vi "Set Aout Cfactor.vi"(8 "error in (no error)":errorcluster, 9 "firmware revision":string(combo), 10 "aout cfactor":T2={"CFactorC (10.0)"=10.0, "CFactorL (100.0)"=100.0}, 11 "VISA resource name":refnum<visa-resource-name>) -> (0 "error out":errorcluster, 2 "bridge error":T1, 3 "VISA resource name out":refnum<visa-resource-name>)   [LabVIEW 2024, in "Andeen-Hagerling 2700A.lvlib"]
doc: "Sets the input to output voltage conversion factor for the\ncapacitance and loss voltage output channels in V/pF and\nV/jpF respectively. This VI gives a direct means of\ncontrolling the sensitivity of the voltage outputs to changes in\nthe DUT."
uses:
  Andeen-Hagerling 2700A.lvlib
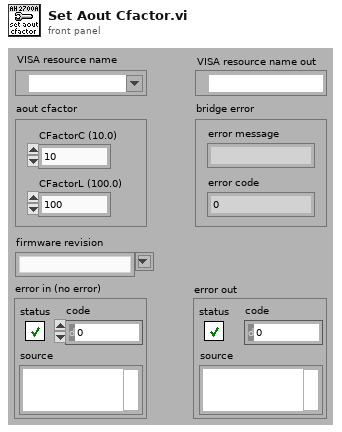
[diagram p1: front panel]
types:
  T1 = cluster{"error message":string, "error code":i32}
  T2 = cluster{"CFactorC (10.0)":dbl, "CFactorL (100.0)":dbl}
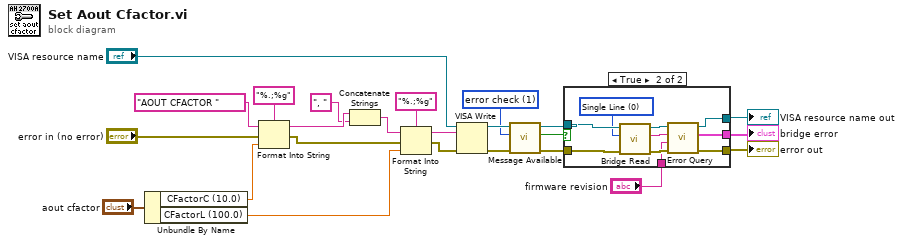
[diagram p0: block diagram]
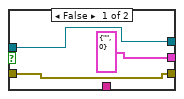
[diagram p2: hidden frame]
diagram:
  w1 = u16 1 items=["none", "error check", "multiline read", "infinite"] ("delay")
  n1 = Unbundle By Name("aout cfactor") -> ("CFactorC (10.0)"=w12:dbl, "CFactorL (100.0)"=w11:dbl)
  n2 = Format Into String(format string="%.;%g", initial string="AOUT CFACTOR " ("command"), error in="error in (no error)", w12) -> (resulting string=w21:string, error out=w22:errorcluster)
  n3 = Concatenate Strings(w21, ", " ("command")) -> (w15:string)
  n4 = Format Into String(format string="%.;%g", initial string=w15, error in=w22, w11) -> (resulting string=w17:string, error out=w18:errorcluster)
  n5 = VISA Write(VISA resource name="VISA resource name", write buffer=w17, error in (no error)=w18) -> (VISA resource name out=w6:refnum<visa-resource-name>, error out=w5:errorcluster)  [unwired: 1 out]
  n6 = call "Message Available.vi"("error in (no error)"=w5, "delay"=w1, "VISA resource name"=w6) -> ("error out"=w8:errorcluster, "message available"=w10:bool, "VISA resource name out"=w9:refnum<visa-resource-name>)  [unwired: 6 in]
  n7 = case shown="True" w10 {
    tunnel: w9 -> [w26 w34]
    tunnel: w8 -> [w27 w33]
    tunnel: "firmware revision" -> [_ w32]
    tunnel: [w27 w31] -> w2
    tunnel: [w26 w30] -> w4
    tunnel: [T1 {"error message"="", "error code"=0} ("bridge error") w29] -> w3
    frame False {
    }
    frame True {
      w28 = u16 0 items=["Single Line", "Multi-Line"] ("Multiline")
      n8 = call "Bridge Read.vi"("error in (no error)"=w33, "multiline"=w28, "VISA resource name"=w34) -> ("error out"=w36:errorcluster, "read buffer"=w37:string, "VISA resource name out"=w35:refnum<visa-resource-name>)  [unwired: 6 in]
      n9 = call "Error Query.vi"("error in (no error)"=w36, "firmware revision"=w32, "measurement line"=w37, "VISA resource name"=w35) -> ("error out"=w31:errorcluster, "bridge error"=w29:T1, "VISA resource name out"=w30:refnum<visa-resource-name>)  [unwired: 5 in]
    }
  }
  "VISA resource name out" <- w4
  "error out" <- w2
  "bridge error" <- w3
